vi "Volume img-Calc frame period.vi"(8 "error in (no error)":errorcluster) -> (0 "error out":errorcluster)   [LabVIEW 2017]
uses:
  Timelapse Viewer/Globals/gl_Time series viewer globals.vi
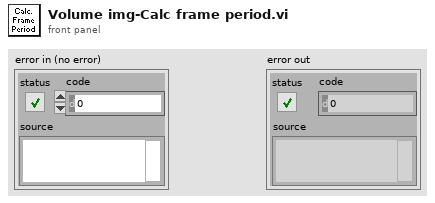
[diagram p1: front panel]
types:
  T1 = typedef "AVI playback header info cluster.ctl" = cluster{"Frame Size":u32, "AOD fill time (us)":dbl, "Dwell time (us)":dbl, "Frame period (ms)":dbl, "Number of Miniscans":u16, "Number of Pixels in Miniscan":u16}
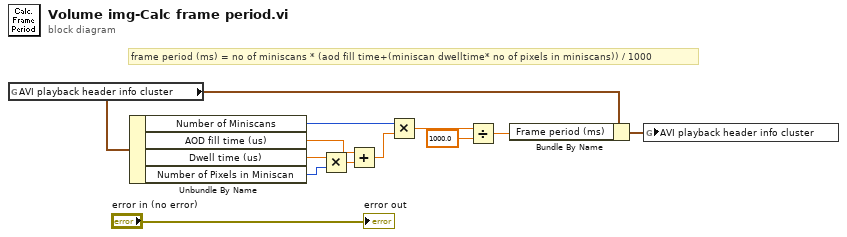
[diagram p0: block diagram]
diagram:
  # "frame period (ms) = no of miniscans * (aod fill time+(miniscan dwelltime* no of pixels in miniscans)) / 1000"
  n1 = global read "gl_Time series viewer globals.vi" "AVI playback header info cluster"() -> (w3:T1)
  n2 = Unbundle By Name(w3) -> ("Number of Miniscans"=w4:u16, "AOD fill time (us)"=w5:dbl, "Dwell time (us)"=w7:dbl, "Number of Pixels in Miniscan"=w8:u16)
  n3 = Multiply(x=w7, y=w8) -> (x*y=w9:dbl)
  n4 = Add(x=w5, y=w9) -> (x+y=w6:dbl)
  n5 = Multiply(x=w4, y=w6) -> (x*y=w10:dbl)
  n6 = Divide(x=w10, y=1000.0) -> (x/y=w12:dbl)
  n7 = Bundle By Name(cluster=w3, "Frame period (ms)"=w12) -> (w2:T1)
  n8 = global write "gl_Time series viewer globals.vi" "AVI playback header info cluster"(w2) -> ()
  "error out" <- "error in (no error)"
